vi "APC_9056_NI9208conf.vi"() -> (0 "Min V out":dbl[](array[numeric])=[-0.02, -0.02, -0.02, -0.02, -0.02, -0.02, -0.02, -0.02, -0.02, -0.02, -0.02, -0.02, -0.02, -0.02, -0.02, -0.02], 1 "Max V out":dbl[](array[numeric])=[0.02, 0.02, 0.02, 0.02, 0.02, 0.02, 0.02, 0.02, 0.02, 0.02, 0.02, 0.02, 0.02, 0.02, 0.02, 0.02], 2 "scaled units out2":string[](array[string])=["kgs", "bar", "bar", "kgs", "kgs", "kgs", "bar", "bar", "bar", "kgs", "bar", "bar", "kgs", "kgs", "kgs", "kgs"], 3 "Y-Intercept out":dbl[](array[numeric]) format="%.2g", 4 "Slope out":dbl[](array[numeric])=[1.0, 1.0, 1.0, 1.0, 1.0, 1.0, 1.0, 1.0, 1.0, 1.0, 1.0, 1.0, 1.0, 1.0, 1.0, 1.0] format="%.2g", 5 "channels name out":string[](array[string])=["NG-FT-001_kgs", "NG-PT-001_bar", "NGDI-PT-001_bar", "O2-FC-001_kgs", "NG-FC-001_kgs", "NGDI-FT-001_kgs", "WF-PT-004_bar", "O2-PT-001_bar", "AR-PT-001_bar", "AR-FT-001_kgs", "WF-PT-016_bar", "WF-PT-014_bar", "SW-FT-001_kgs", "SW-FT-002_kgs", "SW-FT-003_kgs", "SW-FT-004_kgs"])   [LabVIEW 2020]
panel:
  in  "Min I":dbl[](array[numeric])=[-0.02, -0.02, -0.02, -0.02, -0.02, -0.02, -0.02, -0.02, -0.02, -0.02, -0.02, -0.02, -0.02, -0.02, -0.02, -0.02]
  in  "Max I":dbl[](array[numeric])=[0.02, 0.02, 0.02, 0.02, 0.02, 0.02, 0.02, 0.02, 0.02, 0.02, 0.02, 0.02, 0.02, 0.02, 0.02, 0.02]
  in  "scaled units":string[](array[string])=["kgs", "bar", "bar", "kgs", "kgs", "kgs", "bar", "bar", "bar", "kgs", "bar", "bar", "kgs", "kgs", "kgs", "kgs"]
  in  "Y-Intercept":dbl[](array[numeric])=[0.0, 0.0, 0.0, 0.0, 0.0, 0.0, 0.0, 0.0, 0.0, 0.0, 0.0, 0.0, 0.0, 0.0, 0.0, 0.0] format="%.2g"
  in  "Slope":dbl[](array[numeric])=[1.0, 1.0, 1.0, 1.0, 1.0, 1.0, 1.0, 1.0, 1.0, 1.0, 1.0, 1.0, 1.0, 1.0, 1.0, 1.0] format="%.2g"
  in  "channels name":string[](array[string])=["NG-FT-001", "NG-PT-001", "NGDI-PT-001", "O2-FC-001", "NG-FC-001", "NGDI-FT-001", "WF-PT-004", "O2-PT-001", "AR-PT-001", "AR-FT-001", "WF-PT-016", "WF-PT-014", "SW-FT-001", "SW-FT-002", "SW-FT-003", "SW-FT-004"]
  # "NI9208"
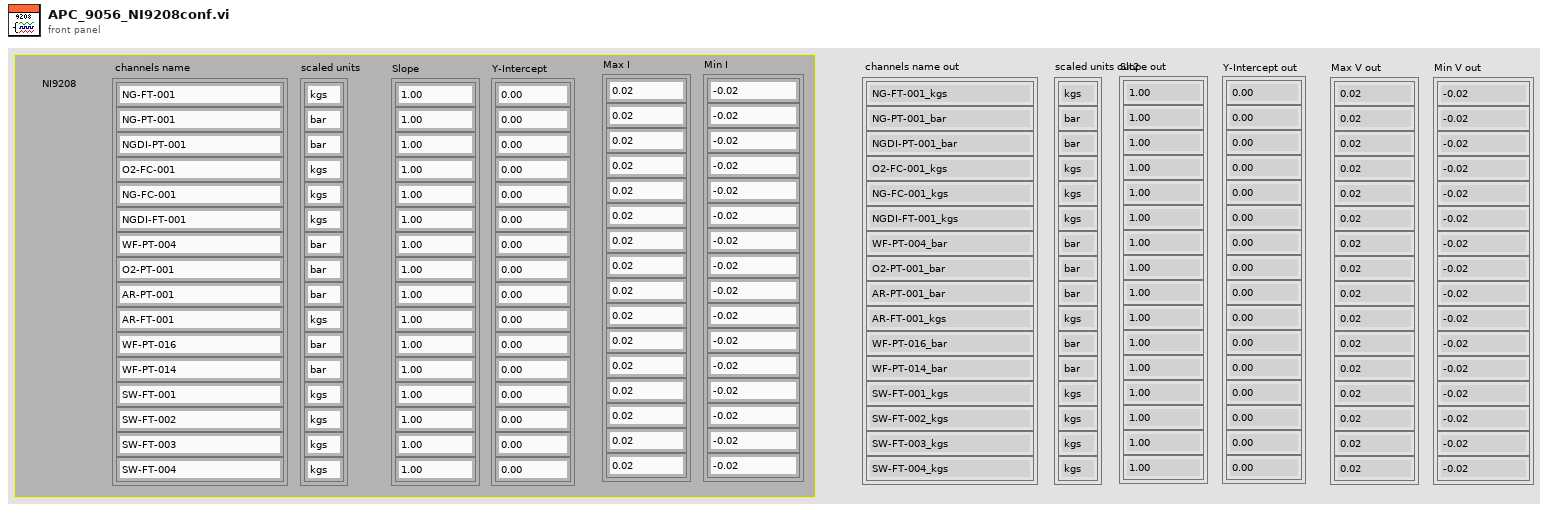
[diagram p1: front panel]
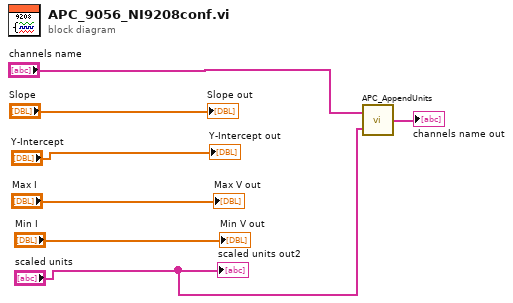
[diagram p0: block diagram]
diagram:
  n1 = call "APC_AppendUnits.vi"("units"="scaled units", "names"="channels name") -> ("names_units"=→"channels name out":string[])
  "Slope out" <- "Slope"
  "Y-Intercept out" <- "Y-Intercept"
  "Max V out" <- "Max I"
  "Min V out" <- "Min I"
  "scaled units out2" <- "scaled units"
